vi "test Import with Parameters Files Missing Something.vi"(8 "error in":errorcluster, 11 "TestCase in":refnum<class "1553 Parameters Import.lvclass">) -> (0 "error out":errorcluster, 3 "TestCase out":refnum<class "1553 Parameters Import.lvclass">)   [LabVIEW 2020, in "1553 Parameters Import.lvclass"]
uses:
  1553 Parameters Import.lvclass
  <vilib>/addons/_JKI Toolkits/VI Tester/TestCase.llb/TestCase.lvclass
  Import/MIL-STD 1553 Import.lvlib
  C:/Program Files (x86)/National Instruments/LabVIEW 2020/vi.lib/addons/_JKI Toolkits/VI Tester/TestCase.llb/TestCase.lvclass
panel:
  out "Array":errorcluster[](array[cluster])
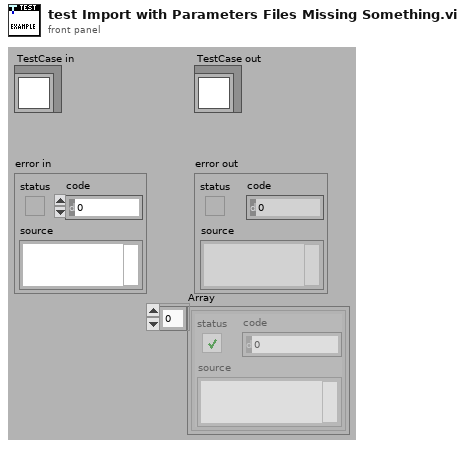
[diagram p1: front panel]
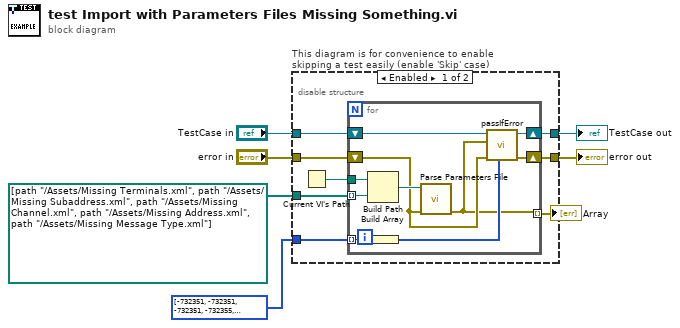
[diagram p0: block diagram]
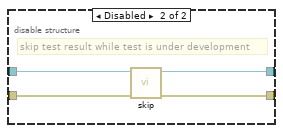
[diagram p2: hidden frame]
diagram:
  n1 = disable-structure "This diagram is for convenience to enable skipping a test easily (enable 'Skip' case)" shown="Enabled" {
    disable-tunnel: "TestCase in" -> [w13 w28]
    disable-tunnel: [w12 w26] -> w3
    disable-tunnel: [w9 w27] -> w5
    disable-tunnel: "error in" -> [w11 w25]
    disable-tunnel: path[] [path "../Assets/Missing Terminals.xml", path "../Assets/Missing Subaddress.xml", path "../Assets/Missing Channel.xml", path "../Assets/Missing Address.xml", path "../Assets/Missing Message Type.xml"] -> [w14 _]
    disable-tunnel: i32[] [-732351, -732351, -732351, -732355, -732351] ("codes") -> [w8 _]
    frame Enabled {
      n2 = Current VI's Path() -> (path=w10:path)
      n3 = for {
        tunnel: w14 -> [w23] mode=indexing
        shift-right: [w20] -> w12
        shift-left: w13 -> [w21]
        shift-right: [w19] -> w9
        shift-left: w11 -> [w18]
        tunnel: w10 -> [w22]
        tunnel: w8 -> [w17] mode=indexing
        tunnel: [w15] -> w7 mode=indexing
        n4 = Build Path(base path=w22, name or relative path=w23) -> (appended path=w24:path)
        n5 = Build Array(w17) -> (w16:i32[])
        n6 = call "Parse Parameters File.vi"("error in"=w18, "path to XML document"=w24) -> ("error out"=w15:errorcluster)  [unwired: 7 in, 2 out]
        n7 = call-dynamic "passIfError.vi"("passing error codes (default = any error code)"=w16, "error in (no error)"=w18, "error"=w15, "TestCase in"=w21) -> ("error out"=w19:errorcluster, "TestCase out"=w20:refnum<class "1553 Parameters Import.lvclass">)  [unwired: 6 in]
      }
      "Array" <- w7
    }
    frame Disabled {
      # "skip test result while test is under development"
      n8 = call <vilib>:"skip.vi"("error in (no error)"=w25, "TestCase in"=w28) -> ("error out"=w27:errorcluster, "TestCase out"=w26:refnum<class "1553 Parameters Import.lvclass">)  [unwired: 8 in]
    }
  }
  "error out" <- w5
  "TestCase out" <- w3
